vi "Send FPGA Telemetry.vi"   [LabVIEW 2014]
uses:
  Session Information.ctl
  FPGA Telemetry.ctl
  Vehicle Status/Subsystem Status.ctl
  Vehicle Status/Subsystem Status Severity.ctl
  Vehicle Status/Subsystem Status Message.ctl
  AIR Status.ctl
  Reason for Shutdown.ctl
  Dash LED Status.ctl
  FPGA/SPI v2/ADXL345 Output.ctl
  Global Data.vi
  <vilib>/FPGAPlugInAG/sbRIO-9626/niLvFpga_Open_sbRIO-9626.vi
  <vilib>/rvi/interface/common/dynamic/niFpgaDynamicAddResources.vi
  <vilib>/Utility/error.llb/Error Cluster From Error Code.vi
  <vilib>/rvi/errors/niLvFpgaAdjustHostInterfaceError.vi
  <vilib>/FPGAPlugInAG/Dynamic/niLvFpga_Close_Dynamic.vi
  <vilib>/rvi/interface/nirviOpenFPGA/nirviOpenFPGA.xnode
  FPGA Bitfiles/Latest.lvbitx
  <vilib>/rvi/interface/nirviReadWriteControl/nirviReadWriteControl.xnode
  <vilib>/rvi/interface/nirviCloseFPGA/nirviCloseFPGA.xnode
  <vilib>/NI_Real-Time Target Support.lvlib
  NiFpgaLv.dll
  <vilib>/rvi/interface/Simulation/niFpgaSimulationCallBeginRW.vi
types:
  T1 = typedef "Session Information.ctl" = cluster{"CLogFilePrefix":string, "CExtraNotes":string, "CCircuit":string, "CCarName":string, "CDriverName":string, "CSessionDescription":string}
  T2 = typedef "FPGA Telemetry.ctl" = cluster{"CPU Load":cluster{"Total (%)":dbl, "Time Critical (%)":dbl, "Timed Structures (%)":dbl, "High (%)":dbl, "Above Normal (%)":dbl, "Normal (%)":dbl, "Background (%)":dbl, "Idle (%)":dbl, "ISR (%)":dbl}, "SVehicleStatus":cluster{"BMS Status":T3, "MC Status":T3, "Shutdown Status":T3, "sbRIO Status":T3, "Vehicle Status":T3, "Shutdown State":enum16{"NI.SC.Initial", "NI.SC.History", "NI.SC.ShallowHistory", "NI.SC.Terminal", "Coolant Pump Started/AIR's On", "AIRs On", "Precharge", "TSMS Off"}, "AIR Status":T6, "Remote Return to Pits":bool, "Reason for Shutdown":T7, "MC State Machine Status":enum16{"NI.SC.Initial", "NI.SC.History", "NI.SC.ShallowHistory", "NI.SC.Terminal", "Broadcast Diag", "Let Current Drop then Disable AIR's", "Enabled", "Disabled"}}, "iPhone HF Data":cluster{"gXiPhone":dbl, "gYiPhone":dbl, "gZiPhone":dbl, "nYawXiPhone":dbl, "nYawYiPhone":dbl, "nYawZiPhone":dbl}, "iPhone LF Data":cluster{"nLatiPhone":dbl, "nLongiPhone":dbl, "nGPSiPhone":dbl}, "stop":bool, "VSupplyOffset":fxp<+,12,4>, "VsbRIOSupply":fxp<+/-,25,6>, "bFPGALED":bool, "TSBRIO":fxp<+/-,33,17>, "rTPS2Unscaled":fxp<+/-,16,1>, "rTPS1Unscaled":fxp<+/-,16,1>, "bTPSConsistent":bool, "bTPSInRange":bool, "rThrottle":fxp<+/-,33,22>, "VTPS2":fxp<+/-,24,5>, "rTPS2":fxp<+/-,31,22>, "VTPS1":fxp<+/-,24,5>, "rTPS1":fxp<+/-,31,22>, "rTPS2Max":fxp<+,16,4>, "rTPS2Min":fxp<+,16,4>, "rTPS1Max":fxp<+,16,4>, "rTPS1Min":fxp<+,16,4>, "bCoolantPumpEnable":bool, "bRTDSEnable":bool, "bTSMSInStatus":bool, "bPosAIREnable":bool, "bBMSOK":bool, "bIMDOK":bool, "bBSPDOK":bool, "bSBRIOOK2":bool, "bSBRIOOK1":bool, "bTSMSOutStatus":bool, "eGreenDash":T8, "eYellowDash":T8, "eRedDash":T8, "bMotorControllerEnable":bool, "tCurrentLap":u32, "bNewLap":bool, "tLastLap":u32, "tLapMin":u32, "V5VSupply":fxp<+/-,24,5>, "bWheelRL":bool, "bWheelRR":bool, "bWheelFR":bool, "bWheelFL":bool, "VBrakePressureR":fxp<+/-,24,5>, "VBrakePressureF":fxp<+/-,24,5>, "bWheelRRStopped":bool, "bWheelRLStopped":bool, "bWheelFRStopped":bool, "bWheelFLStopped":bool, "tWheelRLPeriod":u32, "tWheelRRPeriod":u32, "tWheelFRPeriod":u32, "tWheelFLPeriod":u32, "bBrakeLight":bool, "VShockRR":fxp<+/-,24,5>, "VShockRL":fxp<+/-,24,5>, "VShockFR":fxp<+/-,24,5>, "VShockFL":fxp<+/-,24,5>, "IHighCurrent":fxp<+/-,24,15>, "ILowCurrent":fxp<+/-,24,15>, "pBrakeR":fxp<+,26,13>, "pBrakeF":fxp<+,26,13>, "bHighCurrentOK":bool, "bLowCurrentOK":bool, "bBrakeROK":bool, "bBrakeFOK":bool, "VSteerWheelMiddle":fxp<+/-,26,5>, "aSteerWheel":fxp<+/-,31,13>, "nWheelFL":fxp<+/-,32,16>, "nWheelFR":fxp<+/-,32,16>, "nWheelRL":fxp<+/-,32,16>, "nWheelRR":fxp<+/-,32,16>, "ADXL345 Output":T9, "Tire Diameter(m)":fxp<+,16,1>, "vWheelRR":fxp<+/-,32,18>, "vWheelRL":fxp<+/-,32,18>, "vWheelFR":fxp<+/-,32,18>, "vWheelFL":fxp<+/-,32,18>, "vWheelLowest":fxp<+/-,32,18>, "vWheelHighest":fxp<+/-,32,18>, "bAccel":bool, "vAxleF":fxp<+/-,33,19>, "vCar":fxp<+/-,33,19>, "sLap":fxp<+,32,12>, "rSlipRL":fxp<+/-,12,1>, "rSlipRR":fxp<+/-,12,1>, "rSlipFL":fxp<+/-,12,1>, "rSlipFR":fxp<+/-,12,1>, "NLap":u8, "tLapReference":u32, "tFastestLap":u32}
  T3 = typedef "Subsystem Status.ctl" = cluster{"eStatusSeverity":T4, "NValue":sgl, "CMessage":T5, "bNotOK":bool}
  T4 = typedef "Subsystem Status Severity.ctl" = enum16{"Okay", "Short Warning", "Long Warning", "Return to Pits", "Error", "Danger"}
  T5 = typedef "Subsystem Status Message.ctl" = enum16{"ControllerTemperature", "MotorTemperature", "BatteryTemperature", "BatteryLowVoltage", "LVBattery", "sbRIOTemperature", "Precharge", "BSPD", "IMD", "RemoteReturnToPits", "EStopInterrupted", "NoCellComms", "MCOverSpeed", "MCOverCurrent", "MCOverVoltage", "MCInverterOverTemp", "MCDirectionCommand", "MCInverterTimeout", "MCDesatFault", "MCHWOverCurrent", "MCUnderVoltage", "MCCommandMessageLost", "MotorOverTemp", "MCModAOverTemp", "MCModBOverTemp", "MCModCOverTemp", "MCPCBOverTemp", "MCGateDrv1OverTemp", "MCDateDrv2OverTemp", "MCCurrentSensorFault", "MCResolverNotConnected", "ShutdownLatchTripped", "UnknownBMS", "RemoteEmergency"}
  T6 = typedef "AIR Status.ctl" = enum16{"Off", "Precharge", "On"}
  T7 = typedef "Reason for Shutdown.ctl" = enum16{"None", "BMS", "Shutdown", "sbRIO", "MC", "Remote"}
  T8 = typedef "Dash LED Status.ctl" = enum16{"Off", "Flashing", "On"}
  T9 = typedef "ADXL345 Output.ctl" = cluster{"X":fxp<+/-,14,4>, "Y":fxp<+/-,14,4>, "Z":fxp<+/-,14,4>}
  T10 = typedef "NI_Real-Time Target Support.lvlib/RT CPU Load.ctl" = cluster{"Total (%)":dbl, "Time Critical (%)":dbl, "Timed Structures (%)":dbl, "High (%)":dbl, "Above Normal (%)":dbl, "Normal (%)":dbl, "Background (%)":dbl, "Idle (%)":dbl, "ISR (%)":dbl}
  T11 = typedef "Shutdown State Machine.lvsc/State.ctl" = enum16{"NI.SC.Initial", "NI.SC.History", "NI.SC.ShallowHistory", "NI.SC.Terminal", "Coolant Pump Started/AIR's On", "AIRs On", "Precharge", "TSMS Off"}
  T12 = cluster{"X":fxp<+/-,14,4>, "Y":fxp<+/-,14,4>, "Z":fxp<+/-,14,4>}
  T13 = typedef "MC State Machine.lvsc/State.ctl" = enum16{"NI.SC.Initial", "NI.SC.History", "NI.SC.ShallowHistory", "NI.SC.Terminal", "Broadcast Diag", "Let Current Drop then Disable AIR's", "Enabled", "Disabled"}
  T14 = cluster{"Accel X":dbl, "Accel Y":dbl, "Accel Z":dbl, "Gyro X":dbl, "Gyro Y":dbl, "Gyro Z":dbl}
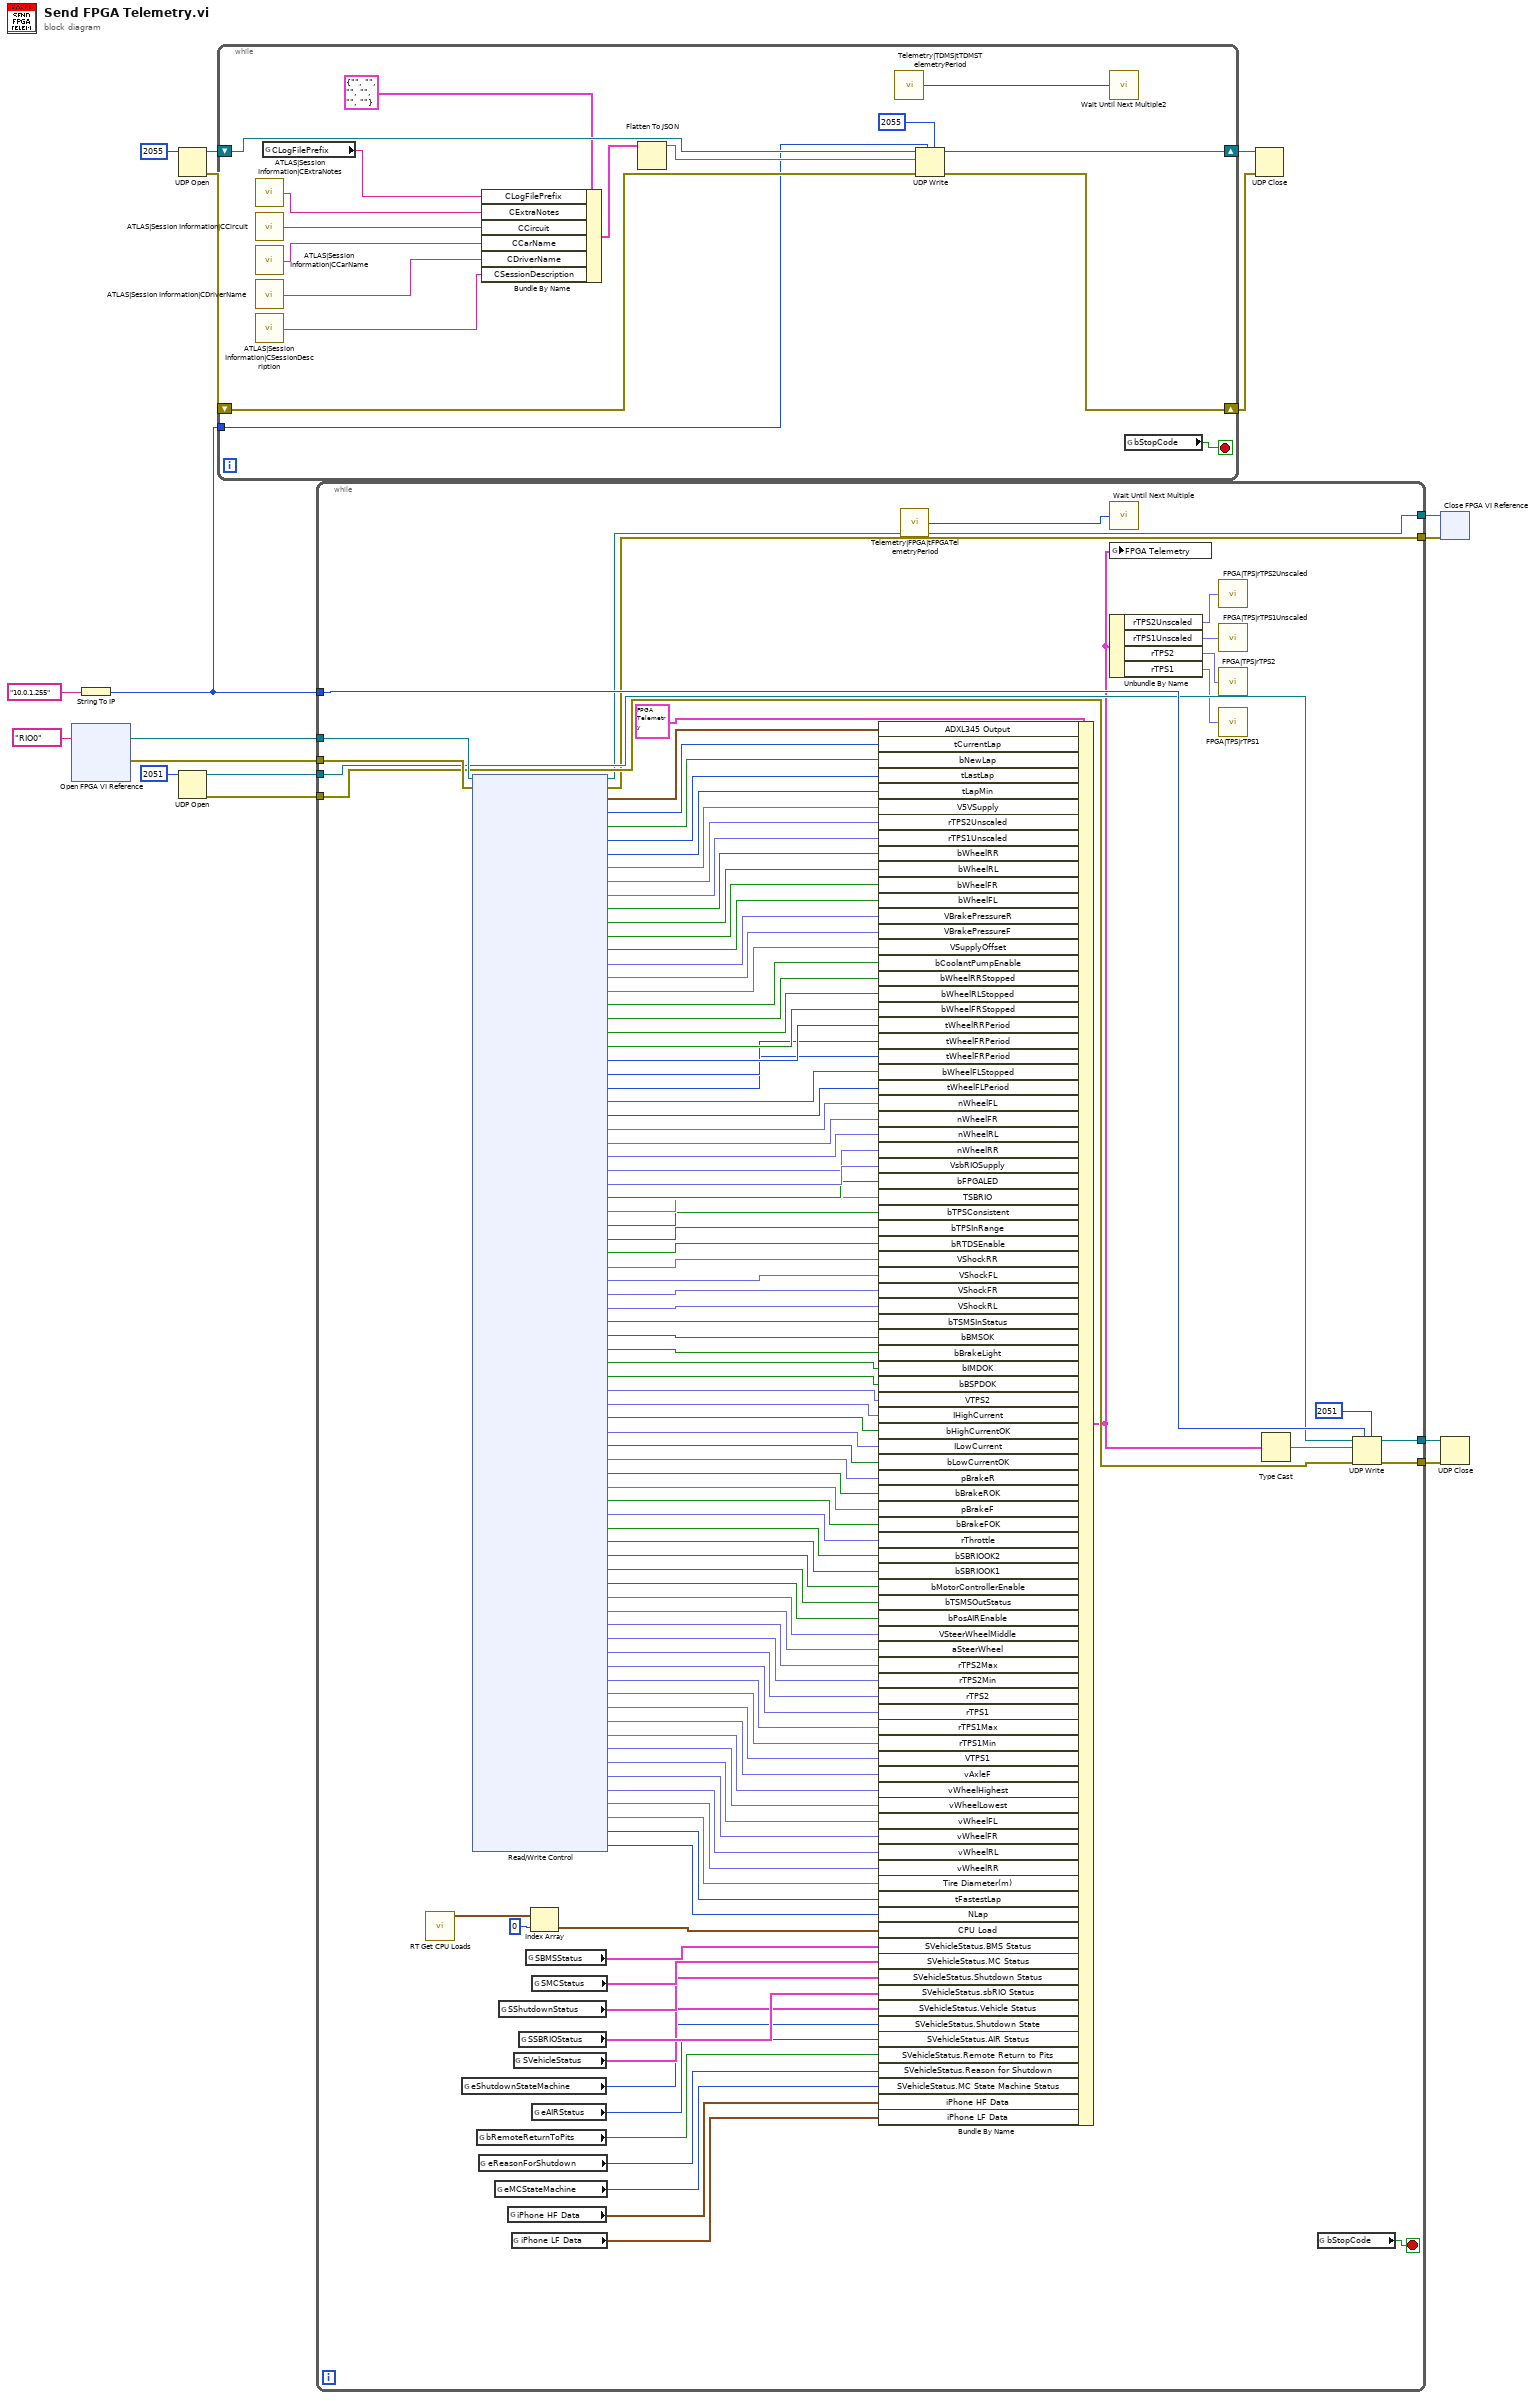
[diagram p0: block diagram]
diagram:
  n1 = xnode "Open FPGA VI Reference"("resource name"=tag "RIO0") -> ("FPGA VI Reference Out"=w17:refnum<k20>, "error out"=w16:errorcluster)  [unwired: 1 in]
  n2 = String To IP(1:"10.0.1.255" ("net address")) -> (0:w5:u32)
  n3 = UDP Open(11:u16 2055 ("port")) -> (port=w7:refnum<k16>, 0:w6:errorcluster)  [unwired: 4 in, 1 out]
  n4 = UDP Open(11:u16 2051 ("port")) -> (port=w10:refnum<k16>, 0:w9:errorcluster)  [unwired: 4 in, 1 out]
  n5 = while {
    tunnel: w5 -> [w30]
    shift-right: [w29] -> w2
    shift-left: w7 -> [w33]
    shift-right: [w28] -> w3
    shift-left: w6 -> [w32]
    stop <- w27 stop-if-true
    n6 = call "ATLAS|Session Information|CExtraNotes"() -> ("Value"=w22:string)
    n7 = call "ATLAS|Session Information|CCircuit"() -> ("Value"=w21:string)
    n8 = call "ATLAS|Session Information|CCarName"() -> ("Value"=w20:string)
    n9 = call "ATLAS|Session Information|CDriverName"() -> ("Value"=w19:string)
    n10 = call "ATLAS|Session Information|CSessionDescription"() -> ("Value"=w18:string)
    n11 = global read "Global Data.vi" "CLogFilePrefix"() -> (w24:string)
    n12 = Bundle By Name(cluster=T1 {"CLogFilePrefix"="", "CExtraNotes"="", "CCircuit"="", "CCarName"="", "CDriverName"="", "CSessionDescription"=""} ("Session Information"), "CLogFilePrefix"=w24, "CExtraNotes"=w22, "CCircuit"=w21, "CCarName"=w20, "CDriverName"=w19, "CSessionDescription"=w18) -> (w23:T1)
    n13 = Flatten To JSON(anything=w23) -> (JSON string=w34:string)  [unwired: 2 in, 1 out]
    n14 = call "Telemetry|TDMS|tTDMSTelemetryPeriod"() -> ("Value"=w26:u32)
    n15 = UDP Write(address=w30, port or service name=u16 2055, connection ID=w33, data in=w34, 8:w32) -> (error out=w28:errorcluster, 3:w29:refnum<k16>)  [unwired: 1 in]
    n16 = call "Wait Until Next Multiple2"("Count(mSec)"=w26) -> ()  [unwired: 1 out]
    n17 = global read "Global Data.vi" "bStopCode"() -> (w27:bool)
  }
  n18 = while {
    tunnel: w17 -> [w145]
    tunnel: w16 -> [w144]
    tunnel: w5 -> [w142]
    tunnel: w10 -> [w140]
    tunnel: w9 -> [w139]
    tunnel: [w138] -> w14
    tunnel: [w137] -> w13
    tunnel: [w136] -> w12
    tunnel: [w135] -> w11
    stop <- w55 stop-if-true
    n19 = call <vilib>:"RT Get CPU Loads.vi"() -> ("CPU loads"=w133:T10[])  [unwired: 10 in, 1 out]
    n20 = global read "Global Data.vi" "eShutdownStateMachine"() -> (w62:T11)
    n21 = xnode "Read/Write Control"("FPGA VI Reference In"=w145, "error in"=w144) -> ("FPGA VI Reference Out"=w136:refnum<k20>, "error out"=w135:errorcluster, "ADXL345 Output"=w131:T12, "tCurrentLap"=w130:u32, "bNewLap"=w129:bool, "tLastLap"=w128:u32, "tLapMin"=w127:u32, "V5VSupply"=w126:fxp<+/-,24,5>, "rTPS2Unscaled"=w125:fxp<+/-,16,1>, "rTPS1Unscaled"=w124:fxp<+/-,16,1>, "bWheelRR"=w123:bool, "bWheelRL"=w122:bool, "bWheelFR"=w121:bool, "bWheelFL"=w120:bool, "VBrakePressureR"=w119:fxp<+/-,24,5>, "VBrakePressureF"=w118:fxp<+/-,24,5>, "VSupplyOffset"=w117:fxp<+,12,4>, "bCoolantPumpEnable"=w116:bool, "bWheelRRStopped"=w115:bool, "bWheelRLStopped"=w114:bool, "bWheelFRStopped"=w113:bool, "tWheelRRPeriod"=w112:u32, "tWheelRLPeriod"=w111:u32, "tWheelFRPeriod"=w110:u32, "bWheelFLStopped"=w109:bool, "tWheelFLPeriod"=w108:u32, "nWheelFL"=w54:fxp<+/-,29,16>, "nWheelFR"=w53:fxp<+/-,29,16>, "nWheelRL"=w52:fxp<+/-,29,16>, "nWheelRR"=w51:fxp<+/-,29,16>, "VsbRIOSupply"=w107:fxp<+/-,25,6>, "bFPGALED"=w106:bool, "TSBRIO"=w105:fxp<+,19,8>, "bTPSConsistent"=w104:bool, "bTPSInRange"=w103:bool, "bRTDSEnable"=w102:bool, "VShockRR"=w101:fxp<+/-,24,5>, "VShockFL"=w100:fxp<+/-,24,5>, "VShockFR"=w99:fxp<+/-,24,5>, "VShockRL"=w98:fxp<+/-,24,5>, "bTSMSInStatus"=w97:bool, "bBMSOK"=w96:bool, "bBrakeLight"=w95:bool, "bIMDOK"=w94:bool, "bBSPDOK"=w93:bool, "VTPS2"=w92:fxp<+/-,24,5>, "IHighCurrent"=w91:fxp<+/-,24,15>, "bHighCurrentOK"=w90:bool, "ILowCurrent"=w89:fxp<+/-,24,15>, "bLowCurrentOK"=w88:bool, "pBrakeR"=w87:fxp<+,26,13>, "bBrakeROK"=w86:bool, "pBrakeF"=w85:fxp<+,26,13>, "bBrakeFOK"=w84:bool, "rThrottle"=w83:fxp<+/-,33,22>, "bSBRIOOK2"=w82:bool, "bSBRIOOK1"=w81:bool, "bMotorControllerEnable"=w80:bool, "bTSMSOutStatus"=w79:bool, "bPosAIREnable"=w78:bool, "VSteerWheelMiddle"=w77:fxp<+/-,26,5>, "aSteerWheel"=w76:fxp<+/-,22,10>, "rTPS2Max"=w75:fxp<+,16,4>, "rTPS2Min"=w74:fxp<+,16,4>, "rTPS2"=w73:fxp<+/-,31,22>, "rTPS1"=w72:fxp<+/-,31,22>, "rTPS1Max"=w71:fxp<+,16,4>, "rTPS1Min"=w70:fxp<+,16,4>, "VTPS1"=w69:fxp<+/-,24,5>, "vAxleF"=w44:fxp<+/-,33,19>, "vWheelHighest"=w43:fxp<+/-,32,18>, "vWheelLowest"=w42:fxp<+/-,32,18>, "vWheelFL"=w41:fxp<+/-,32,18>, "vWheelFR"=w40:fxp<+/-,32,18>, "vWheelRL"=w39:fxp<+/-,32,18>, "vWheelRR"=w38:fxp<+/-,32,18>, "Tire Diameter(m)"=w37:fxp<+,16,1>, "tFastestLap"=w36:u32, "NLap"=w35:u8)
    n22 = global read "Global Data.vi" "bRemoteReturnToPits"() -> (w60:bool)
    n23 = global read "Global Data.vi" "eReasonForShutdown"() -> (w59:T7)
    n24 = global read "Global Data.vi" "eMCStateMachine"() -> (w58:T13)
    n25 = global read "Global Data.vi" "SShutdownStatus"() -> (w65:T3)
    n26 = global read "Global Data.vi" "iPhone HF Data"() -> (w57:T14)
    n27 = global read "Global Data.vi" "iPhone LF Data"() -> (w56:cluster{"Lat":dbl, "Long":dbl, "Speed":dbl})
    n28 = global read "Global Data.vi" "SVehicleStatus"() -> (w63:T3)
    n29 = global read "Global Data.vi" "SSBRIOStatus"() -> (w64:T3)
    n30 = global read "Global Data.vi" "SBMSStatus"() -> (w67:T3)
    n31 = Index Array(array=w133, index=0) -> (element=w68:T10)
    n32 = global read "Global Data.vi" "SMCStatus"() -> (w66:T3)
    n33 = global read "Global Data.vi" "eAIRStatus"() -> (w61:T6)
    n34 = Bundle By Name(cluster=T2 {"CPU Load"={"Total (%)"=0.0, "Time Critical (%)"=0.0, "Timed Structures (%)"=0.0, "High (%)"=0.0, "Above Normal (%)"=0.0, "Normal (%)"=0.0, "Background (%)"=0.0, "Idle (%)"=0.0, "ISR (%)"=0.0}, "SVehicleStatus"={"BMS Status"={"eStatusSeverity"=enum."Okay", "NValue"=0.0, "CMessage"=enum."ControllerTemperature", "bNotOK"=FALSE}, "MC Status"={"eStatusSeverity"=enum."Okay", "NValue"=0.0, "CMessage"=enum."ControllerTemperature", "bNotOK"=FALSE}, "Shutdown Status"={"eStatusSeverity"=enum."Okay", "NValue"=0.0, "CMessage"=enum."ControllerTemperature", "bNotOK"=FALSE}, "sbRIO Status"={"eStatusSeverity"=enum."Okay", "NValue"=0.0, "CMessage"=enum."ControllerTemperature", "bNotOK"=FALSE}, "Vehicle Status"={"eStatusSeverity"=enum."Short Warning", "NValue"=0.0, "CMessage"=enum."ControllerTemperature", "bNotOK"=FALSE}, "Shutdown State"=enum."NI.SC.Initial", "AIR Status"=enum."Off", "Remote Return to Pits"=FALSE, "Reason for Shutdown"=enum."BMS", "MC State Machine Status"=enum."NI.SC.Initial"}, "iPhone HF Data"={"gXiPhone"=0.0, "gYiPhone"=0.0, "gZiPhone"=0.0, "nYawXiPhone"=0.0, "nYawYiPhone"=0.0, "nYawZiPhone"=0.0}, "iPhone LF Data"={"nLatiPhone"=0.0, "nLongiPhone"=0.0, "nGPSiPhone"=0.0}, "stop"=TRUE, "VSupplyOffset"=0.0, "VsbRIOSupply"=0.0, "bFPGALED"=TRUE, "TSBRIO"=0.3482666015625, "rTPS2Unscaled"=0.0, "rTPS1Unscaled"=0.999969482421875, "bTPSConsistent"=FALSE, "bTPSInRange"=FALSE, "rThrottle"=186.34033203125, "VTPS2"=0.0, "rTPS2"=-866.732421875, "VTPS1"=1.0, "rTPS1"=2.0, "rTPS2Max"=0.27001953125, "rTPS2Min"=0.489990234375, "rTPS1Max"=0.6201171875, "rTPS1Min"=0.41015625, "bCoolantPumpEnable"=FALSE, "bRTDSEnable"=FALSE, "bTSMSInStatus"=FALSE, "bPosAIREnable"=FALSE, "bBMSOK"=FALSE, "bIMDOK"=FALSE, "bBSPDOK"=FALSE, "bSBRIOOK2"=FALSE, "bSBRIOOK1"=FALSE, "bTSMSOutStatus"=FALSE, "eGreenDash"=enum."Off", "eYellowDash"=enum."Off", "eRedDash"=enum."Off", "bMotorControllerEnable"=FALSE, "tCurrentLap"=0, "bNewLap"=FALSE, "tLastLap"=0, "tLapMin"=0, "V5VSupply"=0.0, "bWheelRL"=TRUE, "bWheelRR"=TRUE, "bWheelFR"=FALSE, "bWheelFL"=FALSE, "VBrakePressureR"=0.4820976257324219, "VBrakePressureF"=0.4808177947998047, "bWheelRRStopped"=FALSE, "bWheelRLStopped"=FALSE, "bWheelFRStopped"=FALSE, "bWheelFLStopped"=TRUE, "tWheelRLPeriod"=0, "tWheelRRPeriod"=0, "tWheelFRPeriod"=0, "tWheelFLPeriod"=0, "bBrakeLight"=TRUE, "VShockRR"=0.3793773651123047, "VShockRL"=0.3444976806640625, "VShockFR"=0.3425788879394531, "VShockFL"=0.3892974853515625, "IHighCurrent"=-20.724609375, "ILowCurrent"=4.353515625, "pBrakeR"=0.0, "pBrakeF"=0.0, "bHighCurrentOK"=FALSE, "bLowCurrentOK"=FALSE, "bBrakeROK"=FALSE, "bBrakeFOK"=FALSE, "VSteerWheelMiddle"=0.34827280044555664, "aSteerWheel"=124.90449142456055, "nWheelFL"=0.0, "nWheelFR"=0.0, "nWheelRL"=0.0, "nWheelRR"=0.0, "ADXL345 Output"={"X"=0.0, "Y"=0.0, "Z"=0.0}, "Tire Diameter(m)"=0.0, "vWheelRR"=0.0, "vWheelRL"=0.0, "vWheelFR"=0.0, "vWheelFL"=0.0, "vWheelLowest"=0.0, "vWheelHighest"=0.0, "bAccel"=FALSE, "vAxleF"=0.0, "vCar"=0.0, "sLap"=0.0, "rSlipRL"=0.0, "rSlipRR"=0.0, "rSlipFL"=0.0, "rSlipFR"=0.0, "NLap"=0, "tLapReference"=0, "tFastestLap"=0} ("FPGA Telemetry"), "ADXL345 Output"=w131, "tCurrentLap"=w130, "bNewLap"=w129, "tLastLap"=w128, "tLapMin"=w127, "V5VSupply"=w126, "rTPS2Unscaled"=w125, "rTPS1Unscaled"=w124, "bWheelRR"=w123, "bWheelRL"=w122, "bWheelFR"=w121, "bWheelFL"=w120, "VBrakePressureR"=w119, "VBrakePressureF"=w118, "VSupplyOffset"=w117, "bCoolantPumpEnable"=w116, "bWheelRRStopped"=w115, "bWheelRLStopped"=w114, "bWheelFRStopped"=w113, "tWheelRRPeriod"=w112, "tWheelFRPeriod"=w111, "tWheelFRPeriod"=w110, "bWheelFLStopped"=w109, "tWheelFLPeriod"=w108, "nWheelFL"=w54, "nWheelFR"=w53, "nWheelRL"=w52, "nWheelRR"=w51, "VsbRIOSupply"=w107, "bFPGALED"=w106, "TSBRIO"=w105, "bTPSConsistent"=w104, "bTPSInRange"=w103, "bRTDSEnable"=w102, "VShockRR"=w101, "VShockFL"=w100, "VShockFR"=w99, "VShockRL"=w98, "bTSMSInStatus"=w97, "bBMSOK"=w96, "bBrakeLight"=w95, "bIMDOK"=w94, "bBSPDOK"=w93, "VTPS2"=w92, "IHighCurrent"=w91, "bHighCurrentOK"=w90, "ILowCurrent"=w89, "bLowCurrentOK"=w88, "pBrakeR"=w87, "bBrakeROK"=w86, "pBrakeF"=w85, "bBrakeFOK"=w84, "rThrottle"=w83, "bSBRIOOK2"=w82, "bSBRIOOK1"=w81, "bMotorControllerEnable"=w80, "bTSMSOutStatus"=w79, "bPosAIREnable"=w78, "VSteerWheelMiddle"=w77, "aSteerWheel"=w76, "rTPS2Max"=w75, "rTPS2Min"=w74, "rTPS2"=w73, "rTPS1"=w72, "rTPS1Max"=w71, "rTPS1Min"=w70, "VTPS1"=w69, "vAxleF"=w44, "vWheelHighest"=w43, "vWheelLowest"=w42, "vWheelFL"=w41, "vWheelFR"=w40, "vWheelRL"=w39, "vWheelRR"=w38, "Tire Diameter(m)"=w37, "tFastestLap"=w36, "NLap"=w35, "CPU Load"=w68, "SVehicleStatus.BMS Status"=w67, "SVehicleStatus.MC Status"=w66, "SVehicleStatus.Shutdown Status"=w65, "SVehicleStatus.sbRIO Status"=w64, "SVehicleStatus.Vehicle Status"=w63, "SVehicleStatus.Shutdown State"=w62, "SVehicleStatus.AIR Status"=w61, "SVehicleStatus.Remote Return to Pits"=w60, "SVehicleStatus.Reason for Shutdown"=w59, "SVehicleStatus.MC State Machine Status"=w58, "iPhone HF Data"=w57, "iPhone LF Data"=w56) -> (w49:T2)
    n35 = call "Telemetry|FPGA|tFPGATelemetryPeriod"() -> ("Value"=w50:u32)
    n36 = call "Wait Until Next Multiple"("Count(mSec)"=w50) -> ()  [unwired: 1 out]
    n37 = global write "Global Data.vi" "FPGA Telemetry"(w49) -> ()
    n38 = Unbundle By Name(w49) -> ("rTPS2Unscaled"=w48:fxp<+/-,16,1>, "rTPS1Unscaled"=w47:fxp<+/-,16,1>, "rTPS2"=w46:fxp<+/-,31,22>, "rTPS1"=w45:fxp<+/-,31,22>)
    n39 = call "FPGA|TPS|rTPS2Unscaled"("Value"=w48) -> ()
    n40 = call "FPGA|TPS|rTPS1Unscaled"("Value"=w47) -> ()
    n41 = call "FPGA|TPS|rTPS2"("Value"=w46) -> ()
    n42 = call "FPGA|TPS|rTPS1"("Value"=w45) -> ()
    n43 = Type Cast(x=w49) -> (*(type *) &x=w143:string)  [unwired: 1 in]
    n44 = global read "Global Data.vi" "bStopCode"() -> (w55:bool)
    n45 = UDP Write(address=w142, port or service name=u16 2051, connection ID=w140, data in=w143, 8:w139) -> (error out=w137:errorcluster, 3:w138:refnum<k16>)  [unwired: 1 in]
  }
  n46 = UDP Close(connection ID=w2, 8:w3) -> ()  [unwired: 2 out]
  n47 = xnode "Close FPGA VI Reference"("FPGA VI Reference In"=w12, "error in"=w11) -> ()  [unwired: 1 out]
  n48 = UDP Close(connection ID=w14, 8:w13) -> ()  [unwired: 2 out]
